vi "Group Selection List By Row.vi"(8 "error in (no error)":errorcluster, 10 "Pixel Tolerance between rows (20)":i32=20, 11 "Parsed Selection List":T1[](array[typedef])) -> (0 "error out":errorcluster, 3 "Parsed Selection List (Geographic Rows)":cluster{"Selection List":T1[]}[](array[cluster]))   [LabVIEW 2016]
uses:
  <resource>/dialog/QuickDrop/plugins/_WireMultipleSupport/Node Terminal Info.ctl
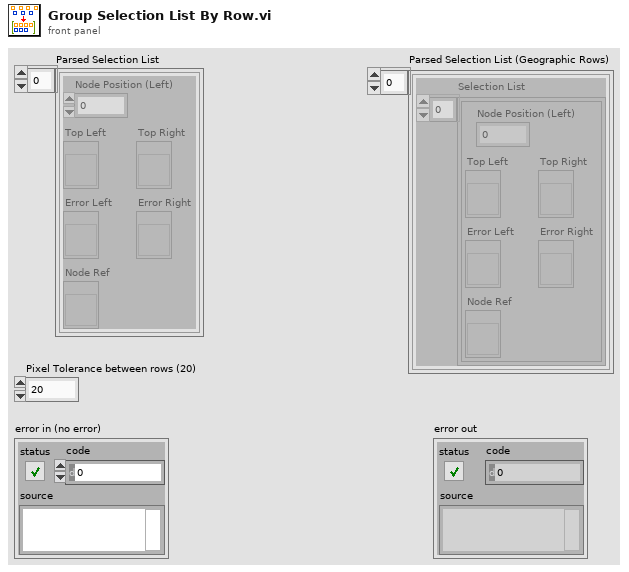
[diagram p1: front panel]
types:
  T1 = typedef "Node Terminal Info.ctl" = cluster{"Node Position (Left)":i32, "Node Ref":refnum<vi>, "Top Left":refnum<vi>, "Top Right":refnum<vi>, "Error Left":refnum<vi>, "Error Right":refnum<vi>}
  T2 = typedef "LVRectTypeDef.ctl" = cluster{"Left":i16, "Top":i16, "Right":i16, "Bottom":i16}
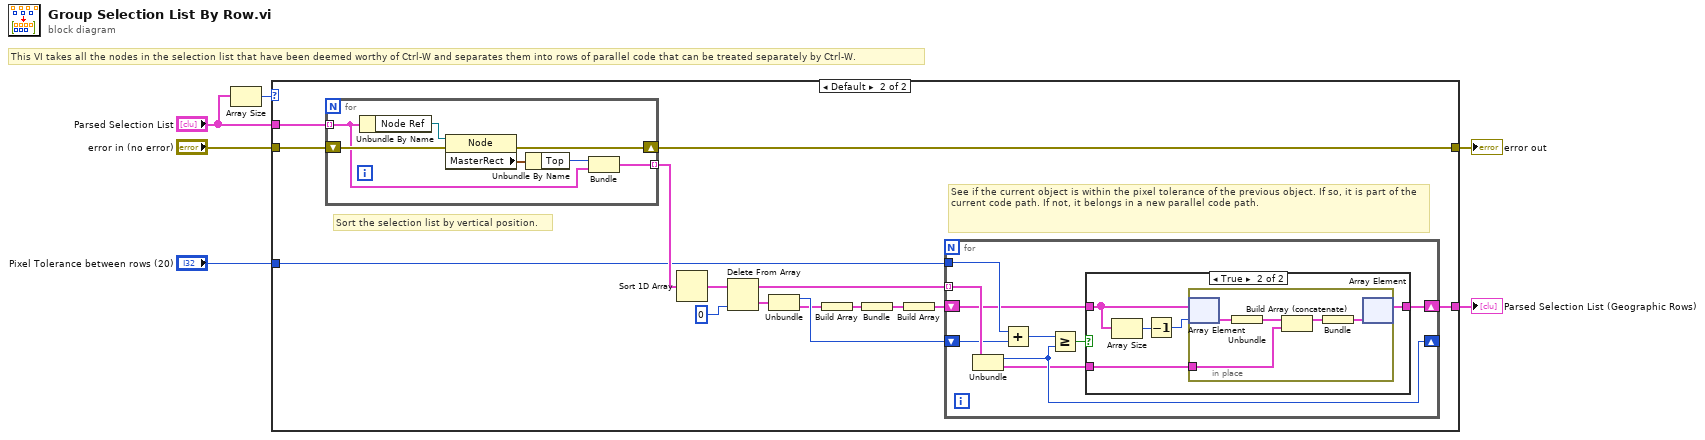
[diagram p0: block diagram]
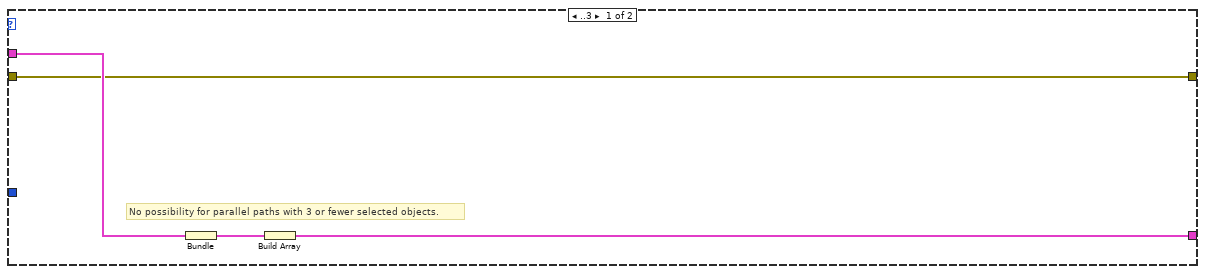
[diagram p2: hidden frame]
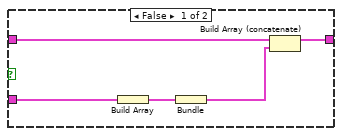
[diagram p3: hidden frame]
diagram:
  # "This VI takes all the nodes in the selection list that have been deemed worthy of Ctrl-W and separates them into rows of parallel code that can be treated separately by Ctrl-W."
  n1 = Array Size(array="Parsed Selection List") -> (size(s)=w2:i32)
  n2 = case shown="Default" w2 {
    tunnel: [w7 w23] -> w6
    tunnel: [w8 w22] -> w5
    tunnel: "Pixel Tolerance between rows (20)" -> [_ w13]
    tunnel: "Parsed Selection List" -> [w10 w12]
    tunnel: "error in (no error)" -> [w7 w25]
    frame ..3 {
      # "No possibility for parallel paths with 3 or fewer selected objects."
      n3 = Bundle("Parsed Selection List"=w10) -> (w9:cluster{"Parsed Selection List":T1[]})  [unwired: 1 in]
      n4 = Build Array(w9) -> (w8:cluster{"Parsed Selection List":T1[]}[])
    }
    frame Default {
      # "See if the current object is within the pixel tolerance of the previous object. If so, it is part of the current code path. If not, it belongs in a new parallel code path."
      # "Sort the selection list by vertical position."
      n5 = for {
        tunnel: w12 -> [w50] mode=indexing
        shift-right: [w55] -> w23
        shift-left: w25 -> [w56]
        tunnel: [w54] -> w24 mode=indexing
        n6 = Unbundle By Name(w50) -> ("Node Ref"=w51:refnum<vi>)
        n7 = property class="Node"(reference=w51, error in=w56) -> (error out=w55:errorcluster, "MasterRect"=w53:T2)  [unwired: 1 out]
        n8 = Unbundle By Name(w53) -> ("Top"=w52:i16)
        n9 = Bundle("Top"=w52, "cluster"=w50) -> (w54:cluster{"Top":i16, "cluster":T1})  [unwired: 1 in]
      }
      n10 = Sort 1D Array(array=w24) -> (sorted array=w21:cluster{"Top":i16, "cluster":T1}[])
      n11 = Delete From Array(array=w21, index=0) -> (deleted portion=w19:cluster{"Top":i16, "cluster":T1}, array with subset deleted=w20:cluster{"Top":i16, "cluster":T1}[])  [unwired: 1 in]
      n12 = Unbundle(w19) -> ("Top"=w18:i16, "cluster"=w17:T1)
      n13 = Build Array(w17) -> (w16:T1[])
      n14 = Bundle(w16) -> (w15:cluster{T1[]})  [unwired: 1 in]
      n15 = Build Array(w15) -> (w14:cluster{T1[]}[])
      n16 = for {
        tunnel: w20 -> [w34] mode=indexing
        shift-right: [w26] -> w22
        shift-left: w14 -> [w27]
        shift-right: [w30] -> _
        shift-left: w18 -> [w33]
        tunnel: w13 -> [w31]
        n17 = Unbundle(w34) -> ("Top"=w30:i16, "cluster"=w28:T1)
        n18 = Add(x=w31, y=w33) -> (x+y=w32:i32)
        n19 = Greater Or Equal?(x=w32, y=w30) -> (x >= y?=w29:bool)
        n20 = case shown="True" w29 {
          tunnel: w28 -> [w38 w41]
          tunnel: w27 -> [w37 w43]
          tunnel: [w35 w40] -> w26
          frame False {
            n21 = Build Array(w38) -> (w39:T1[])
            n22 = Bundle(w39) -> (w36:cluster{T1[]})  [unwired: 1 in]
            n23 = Build Array (concatenate)(w37, w36) -> (w35:cluster{T1[]}[])
          }
          frame True {
            n24 = Array Size(array=w43) -> (size(s)=w44:i32)
            n25 = Decrement(x=w44) -> (x-1=w42:i32)
            n26 = in-place {
              in-place-border: w41 -> [w47]
              n27 = in-place-array #1(w43, w42) -> (w49:cluster{T1[]})
              n28 = Unbundle(w49) -> (w48:T1[])
              n29 = Build Array (concatenate)(w48, w47) -> (w46:T1[])
              n30 = Bundle(w46) -> (w45:cluster{T1[]})  [unwired: 1 in]
              n31 = in-place-array #1(w45) -> (w40:cluster{T1[]}[])  [unwired: 1 out]
            }
          }
        }
      }
    }
  }
  "error out" <- w6
  "Parsed Selection List (Geographic Rows)" <- w5
